vi "串口操作.vi"(0 "VISA资源名称":refnum<visa-resource-name>, 1 "是否需要清空缓冲区？":bool, 2 "Mask":T1=16 items=["清空接收缓冲区"=16, "向设备写入传输缓冲区"=32, "清空接收缓冲区（无I/O）"=64, "清空传输缓冲区"=128], 3 "是否有协议？":bool, 4 "写入指令":string, 5 "错误输入（无错误）":errorcluster, 6 "读取时间":u32) -> (14 "VISA资源名称输出":refnum<visa-resource-name>, 15 "读取数据":string, 19 "错误输出":errorcluster)   [LabVIEW 2017]
uses:
  <vilib>/Instr/_visa.llb/VISA Flush IO Buffer Mask.ctl
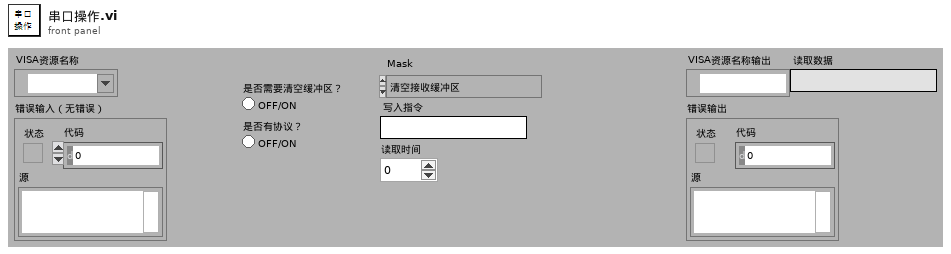
[diagram p1: front panel]
types:
  T1 = typedef "VISA Flush IO Buffer Mask.ctl" = u16
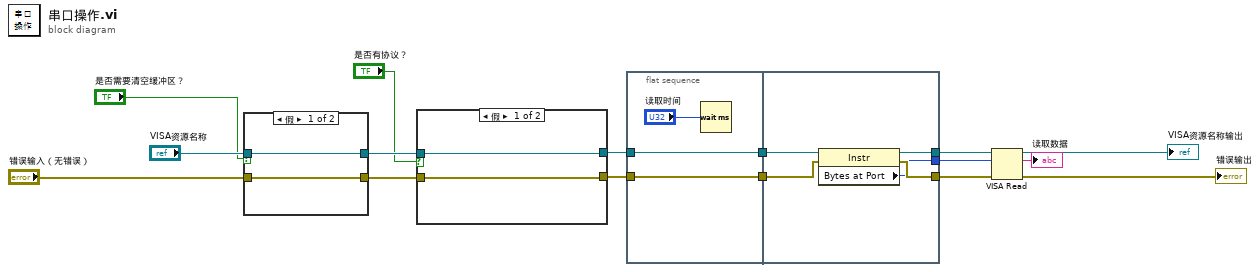
[diagram p0: block diagram]
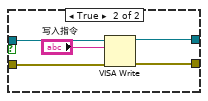
[diagram p2: hidden frame]
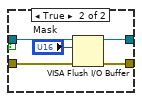
[diagram p3: hidden frame]
diagram:
  n1 = case shown="假" "是否需要清空缓冲区？" {
    tunnel: [w18 w23] -> w16
    tunnel: "VISA资源名称" -> [w18 w22]
    tunnel: "错误输入（无错误）" -> [w17 w21]
    tunnel: [w17 w19] -> w12
    frame False {
    }
    frame True {
      n2 = VISA Flush I/O Buffer(VISA resource name=w22, mask (16)="Mask", error in (no error)=w21) -> (VISA resource name out=w23:refnum<visa-resource-name>, error out=w19:errorcluster)
    }
  }
  n3 = case shown="假" "是否有协议？" {
    tunnel: w16 -> [w25 w30]
    tunnel: w12 -> [w24 w29]
    tunnel: [w25 w27] -> w9
    tunnel: [w24 w26] -> w7
    frame False {
    }
    frame True {
      n4 = VISA Write(VISA resource name=w30, write buffer="写入指令", error in (no error)=w29) -> (VISA resource name out=w27:refnum<visa-resource-name>, error out=w26:errorcluster)  [unwired: 1 out]
    }
  }
  n5 = flat-sequence {
    tunnel: [w32] -> w10
    tunnel: w9 -> [w32]
    tunnel: [w31] -> w8
    tunnel: w7 -> [w31]
    tunnel: w10 -> [w38]
    tunnel: w8 -> [w37]
    tunnel: [w36] -> w6
    tunnel: [w35] -> w5
    tunnel: [w34] -> w4
    frame #0 {
      n6 = Wait (ms)(milliseconds to wait="读取时间") -> ()  [unwired: 1 out]
    }
    frame #1 {
      n7 = property class="Instr"(reference=w38, error in=w37) -> (reference out=w36:refnum<visa-resource-name>, error out=w35:errorcluster, "Bytes at Port"=w34:u32)
    }
  }
  n8 = VISA Read(VISA resource name=w6, byte count=w4, error in (no error)=w5) -> (VISA resource name out=→"VISA资源名称输出":refnum<visa-resource-name>, read buffer=→"读取数据":string, error out=→"错误输出":errorcluster)  [unwired: 1 out]
